vi "Parse U64 Ctl Regs.vi"(9 "NTeeths In":T5, 10 "FullyCustomTeeths In":T3, 11 "U64":T1[](array[typedef])) -> (1 "NTeeths Out":T5, 2 "FullyCustomTeeths In":T3)   [LabVIEW 2011, in "Engine Sim System Explorer.lvlib"]
uses:
  Engine Sim System Explorer.lvlib
  TypeDefs/NTeethRegs.ctl
  TypeDefs/FullyCustomRegs.ctl
  <userlib>/_FPGA Interface Advanced Tools/FPGA Bitfile Utility/TypeDefs/Scalar Register.ctl
  <userlib>/_FPGA Interface Advanced Tools/FPGA Bitfile Utility/FPGA Bitfile Utility.lvlib
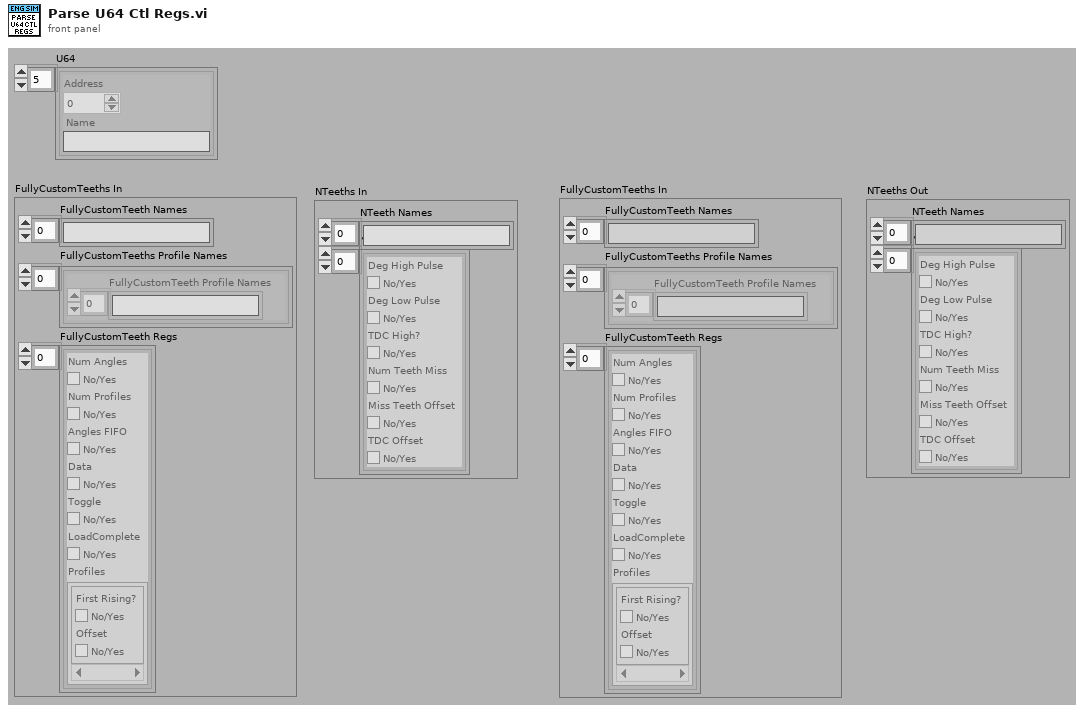
[diagram p1: front panel]
types:
  T1 = typedef "FPGA Bitfile Utility.lvlib/Scalar Register.ctl" = cluster{"Address":u32, "Name":string}
  T2 = typedef "Engine Sim System Explorer.lvlib/FullyCustomRegs.ctl" = cluster{"Num Angles":bool, "Num Profiles":bool, "Angles FIFO":bool, "Data":bool, "Toggle":bool, "LoadComplete":bool, "Profiles":cluster{"First Rising?":bool, "Offset":bool}[]}
  T3 = cluster{"FullyCustomTeeth Names":string[], "FullyCustomTeeths Profile Names":cluster{"FullyCustomTeeth Profile Names":string[]}[], "FullyCustomTeeth Regs":T2[]}
  T4 = typedef "Engine Sim System Explorer.lvlib/NTeethRegs.ctl" = cluster{"Deg High Pulse":bool, "Deg Low Pulse":bool, "TDC High?":bool, "Num Teeth Miss":bool, "Miss Teeth Offset":bool, "TDC Offset":bool}
  T5 = cluster{"NTeeth Names":string[], "NTeeth Regs":T4[]}
  T6 = cluster{"FullyCustomTeeth Profile Names":string[]}
  T7 = cluster{"FullyCustomTeeth Profile Names":string[]}[]
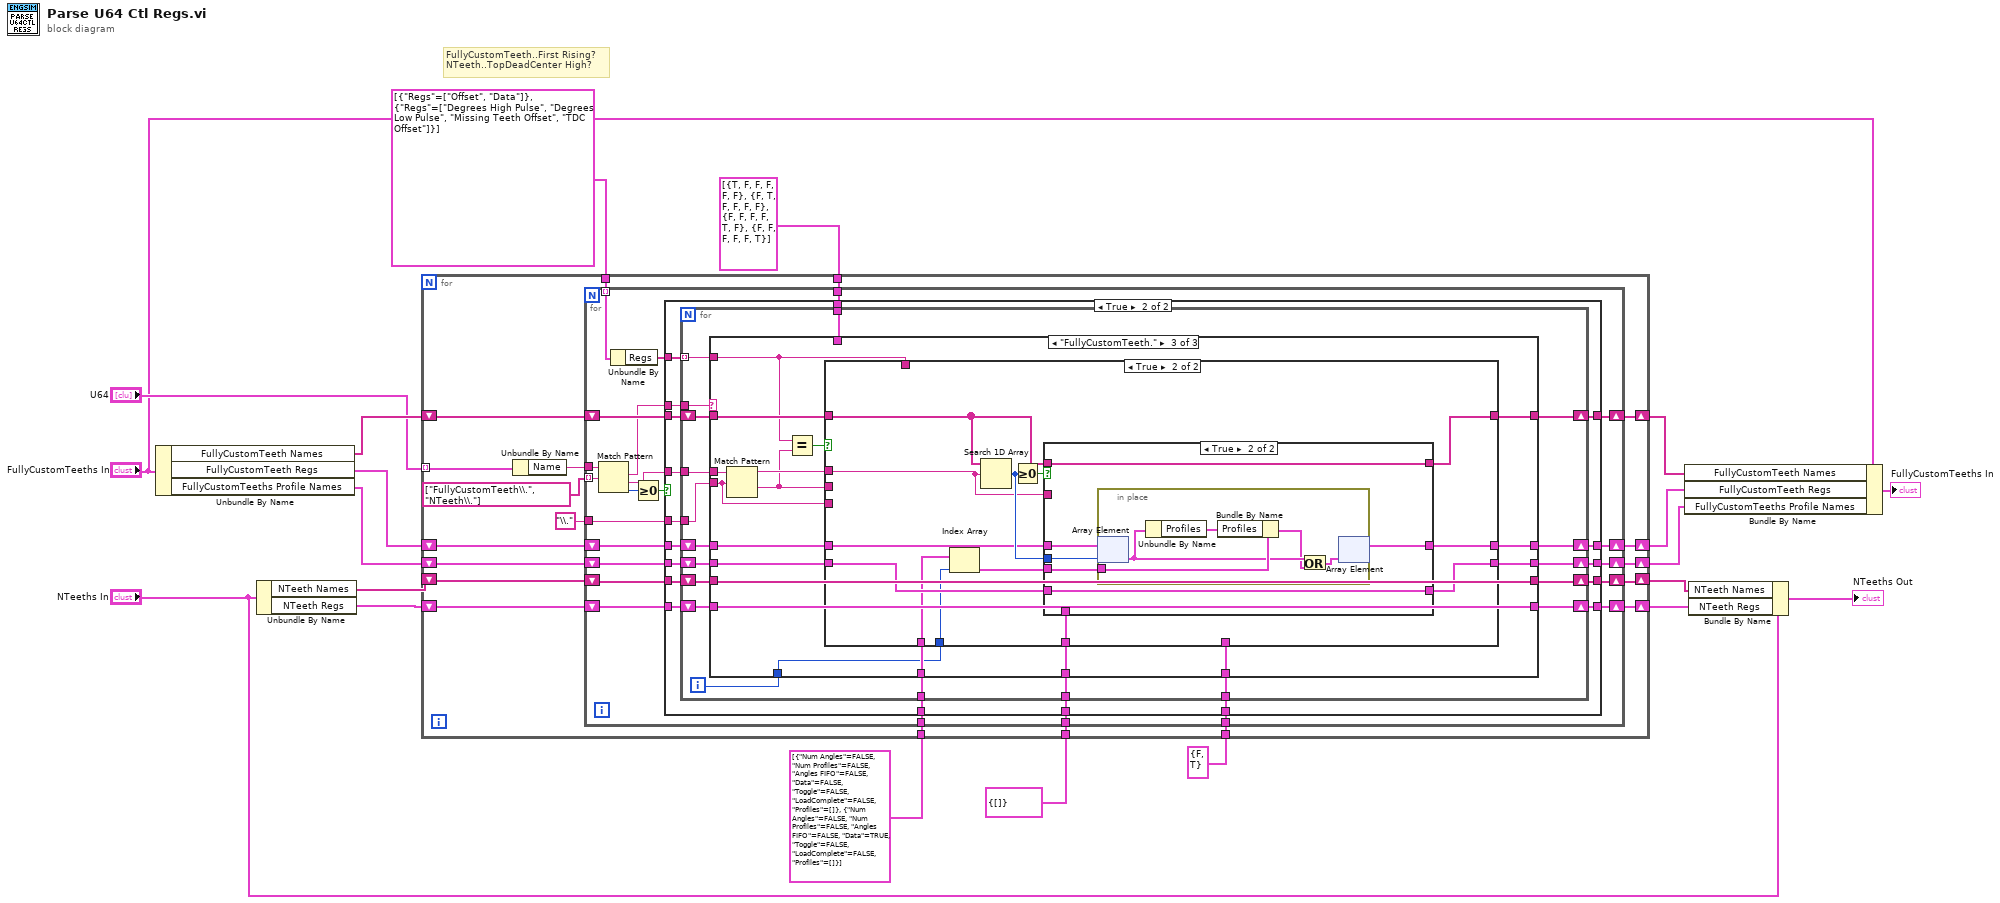
[diagram p0: block diagram]
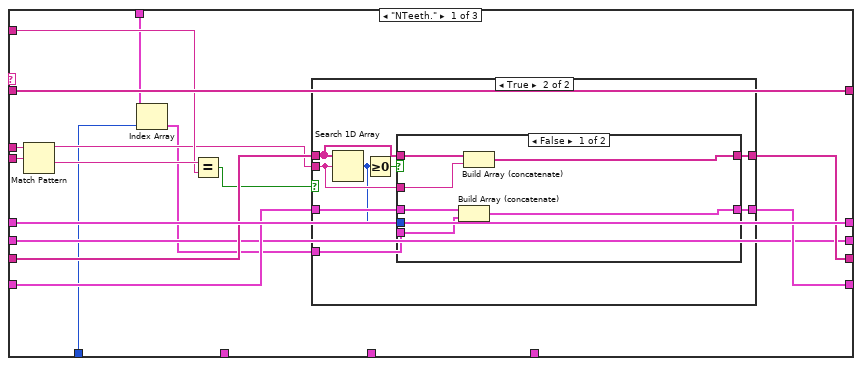
[diagram p3: hidden frame]
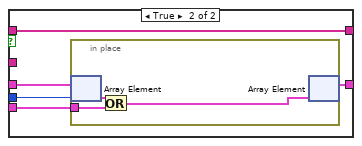
[diagram p5: hidden frame]
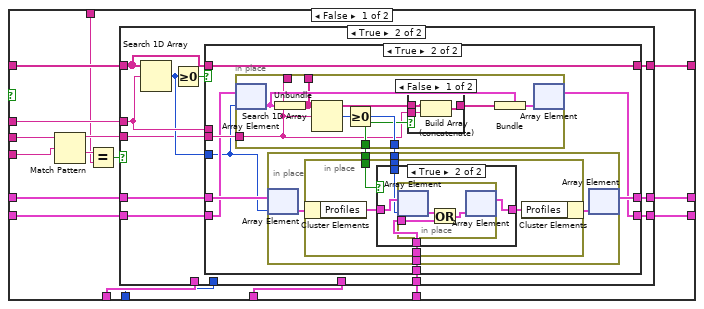
[diagram p7: hidden frame]
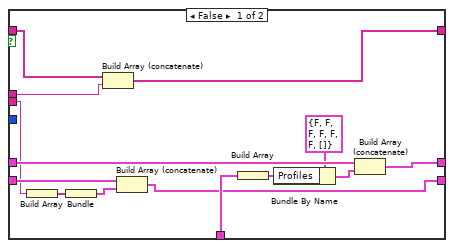
[diagram p9: hidden frame]
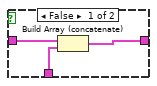
[diagram p11: hidden frame]
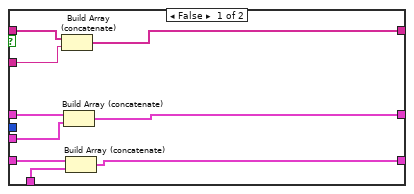
[diagram p12: hidden frame]
diagram:
  # "FullyCustomTeeth..First Rising?\nNTeeth..TopDeadCenter High?"
  n1 = Unbundle By Name("FullyCustomTeeths In") -> ("FullyCustomTeeth Names"=w12:string[], "FullyCustomTeeth Regs"=w13:T2[], "FullyCustomTeeths Profile Names"=w5:T7)
  n2 = Unbundle By Name("NTeeths In") -> ("NTeeth Names"=w14:string[], "NTeeth Regs"=w15:T4[])
  n3 = for {
    tunnel: "U64" -> [w39] mode=indexing
    tunnel: cluster{"First Rising?":bool, "Offset":bool} {"First Rising?"=FALSE, "Offset"=TRUE} ("Profile") -> [w37]
    shift-right: [w36] -> w17
    shift-left: w13 -> [w35]
    shift-right: [w34] -> w16
    shift-left: w12 -> [w33]
    tunnel: cluster{"Regs":string[]}[] [{"Regs"=["Offset", "Data"]}, {"Regs"=["Degrees High Pulse", "Degrees Low Pulse", "Missing Teeth Offset", "TDC Offset"]}] -> [w31]
    shift-right: [w30] -> w20
    shift-left: w15 -> [w29]
    tunnel: T4[] [{"Deg High Pulse"=TRUE, "Deg Low Pulse"=FALSE, "TDC High?"=FALSE, "Num Teeth Miss"=FALSE, "Miss Teeth Offset"=FALSE, "TDC Offset"=FALSE}, {"Deg High Pulse"=FALSE, "Deg Low Pulse"=TRUE, "TDC High?"=FALSE, "Num Teeth Miss"=FALSE, "Miss Teeth Offset"=FALSE, "TDC Offset"=FALSE}, {"Deg High Pulse"=FALSE, "Deg Low Pulse"=FALSE, "TDC High?"=FALSE, "Num Teeth Miss"=FALSE, "Miss Teeth Offset"=TRUE, "TDC Offset"=FALSE}, {"Deg High Pulse"=FALSE, "Deg Low Pulse"=FALSE, "TDC High?"=FALSE, "Num Teeth Miss"=FALSE, "Miss Teeth Offset"=FALSE, "TDC Offset"=TRUE}] -> [w28]
    shift-right: [w26] -> w19
    shift-left: w14 -> [w25]
    shift-right: [w23] -> w4
    shift-left: w5 -> [w24]
    tunnel: T2[] [{"Num Angles"=FALSE, "Num Profiles"=FALSE, "Angles FIFO"=FALSE, "Data"=FALSE, "Toggle"=FALSE, "LoadComplete"=FALSE, "Profiles"=[]}, {"Num Angles"=FALSE, "Num Profiles"=FALSE, "Angles FIFO"=FALSE, "Data"=TRUE, "Toggle"=FALSE, "LoadComplete"=FALSE, "Profiles"=[]}] -> [w22]
    tunnel: T6 {"FullyCustomTeeth Profile Names"=[]} ("FullyCustomTeeth") -> [w21]
    n4 = Unbundle By Name(w39) -> ("Name"=w38:string)
    n5 = for {
      tunnel: w38 -> [w62]
      tunnel: w37 -> [w58]
      tunnel: string[] ["FullyCustomTeeth\\.", "NTeeth\\."] -> [w53] mode=indexing
      shift-right: [w55] -> w34
      shift-left: w33 -> [w54]
      shift-right: [w57] -> w36
      shift-left: w35 -> [w56]
      tunnel: w31 -> [w52] mode=indexing
      shift-right: [w49] -> w30
      shift-left: w29 -> [w48]
      tunnel: w28 -> [w47]
      tunnel: "\\." ("regular expression") -> [w46]
      shift-right: [w45] -> w26
      shift-left: w25 -> [w44]
      shift-right: [w42] -> w23
      shift-left: w24 -> [w43]
      tunnel: w22 -> [w41]
      tunnel: w21 -> [w40]
      n6 = Match Pattern(string=w62, regular expression=w53) -> (match substring=w50:string, after substring=w59:string, offset past match=w61:i32)  [unwired: 1 in, 1 out]
      n7 = Unbundle By Name(w52) -> ("Regs"=w51:string[])
      n8 = Greater Or Equal To 0?(x=w61) -> (x >= 0?=w60:bool)
      n9 = case shown="True" w60 {
        tunnel: w59 -> [_ w85]
        tunnel: w58 -> [_ w84]
        tunnel: [w66 w83] -> w57
        tunnel: w56 -> [w66 w82]
        tunnel: [w67 w81] -> w55
        tunnel: w54 -> [w67 w80]
        tunnel: w51 -> [_ w79]
        tunnel: w50 -> [_ w78]
        tunnel: [w65 w77] -> w49
        tunnel: w48 -> [w65 w76]
        tunnel: w47 -> [_ w75]
        tunnel: w46 -> [_ w74]
        tunnel: [w64 w73] -> w45
        tunnel: w44 -> [w64 w72]
        tunnel: w43 -> [w63 w71]
        tunnel: [w63 w70] -> w42
        tunnel: w41 -> [_ w69]
        tunnel: w40 -> [_ w68]
        frame False {
        }
        frame True {
          n10 = for {
            tunnel: w85 -> [w93]
            tunnel: w84 -> [w104]
            shift-right: [w101] -> w81
            shift-left: w80 -> [w100]
            shift-right: [w103] -> w83
            shift-left: w82 -> [w102]
            tunnel: w79 -> [w91] mode=indexing
            tunnel: w78 -> [w99]
            shift-right: [w98] -> w77
            shift-left: w76 -> [w96]
            tunnel: w75 -> [w97]
            tunnel: w74 -> [w92]
            shift-right: [w95] -> w73
            shift-left: w72 -> [w94]
            shift-right: [w89] -> w70
            shift-left: w71 -> [w90]
            tunnel: w69 -> [w88]
            tunnel: w68 -> [w87]
            i -> [w86]
            n11 = case shown="\"FullyCustomTeeth.\"" w99 {
              tunnel: w93 -> [w113 _ w160]
              tunnel: w104 -> [_ _ w167]
              tunnel: [w119 w148 w166] -> w103
              tunnel: w102 -> [w119 w148 w165]
              tunnel: [w120 w149 w164] -> w101
              tunnel: w100 -> [w120 w149 w163]
              tunnel: [w116 w147 w162] -> w98
              tunnel: w97 -> [w107 _ _]
              tunnel: w96 -> [w115 w147 w162]
              tunnel: [w117 w146 w161] -> w95
              tunnel: w94 -> [w118 w146 w161]
              tunnel: w92 -> [w112 _ w159]
              tunnel: w91 -> [w111 _ w153]
              tunnel: w90 -> [w108 w145 w157]
              tunnel: [w108 w145 w156] -> w89
              tunnel: w88 -> [_ _ w152]
              tunnel: w87 -> [_ _ w151]
              tunnel: w86 -> [w106 _ w150]
              frame "NTeeth." {
                n12 = Match Pattern(string=w113, regular expression=w112) -> (before substring=w109:string, after substring=w114:string)  [unwired: 1 in, 2 out]
                n13 = Index Array(array=w107, index=w106) -> (element=w105:T4)
                n14 = Equal?(x=w114, y=w111) -> (x = y?=w110:bool)
                n15 = case shown="True" w110 {
                  tunnel: w109 -> [_ w126]
                  tunnel: [w121 w128] -> w116
                  tunnel: w115 -> [w121 w129]
                  tunnel: [w122 w125] -> w117
                  tunnel: w118 -> [w122 w127]
                  tunnel: w105 -> [_ w123]
                  frame False {
                  }
                  frame True {
                    n16 = Search 1D Array(1D array=w127, element=w126) -> (index of element=w124:i32)  [unwired: 1 in]
                    n17 = Greater Or Equal To 0?(x=w124) -> (x >= 0?=w130:bool)
                    n18 = case shown="False" w130 {
                      tunnel: w129 -> [w136 w140]
                      tunnel: w123 -> [w135 w138]
                      tunnel: [w134 w137] -> w128
                      tunnel: w127 -> [w133 w141]
                      tunnel: w126 -> [w132 _]
                      tunnel: [w131 w141] -> w125
                      tunnel: w124 -> [_ w139]
                      frame False {
                        n19 = Build Array (concatenate)(w136, w135) -> (w134:T4[])
                        n20 = Build Array (concatenate)(w133, w132) -> (w131:string[])
                      }
                      frame True {
                        n21 = in-place {
                          in-place-border: w138 -> [w143]
                          n22 = in-place-array #1(w140, w139) -> (w144:T4)
                          n23 = Or(x=w144, y=w143) -> (x .or. y?=w142:T4)
                          n24 = in-place-array #1(w142) -> (w137:T4[])  [unwired: 1 out]
                        }
                      }
                    }
                  }
                }
              }
              frame Default {
              }
              frame "FullyCustomTeeth." {
                n25 = Match Pattern(string=w160, regular expression=w159) -> (before substring=w158:string, after substring=w154:string)  [unwired: 1 in, 2 out]
                n26 = Equal?(x=w153, y=w154) -> (x = y?=w155:bool)
                n27 = case shown="True" w155 {
                  tunnel: w167 -> [w184 _]
                  tunnel: [w183 w258] -> w166
                  tunnel: w165 -> [w182 w261]
                  tunnel: [w181 w259] -> w164
                  tunnel: w163 -> [w180 w264]
                  tunnel: w154 -> [w179 _]
                  tunnel: w159 -> [w178 _]
                  tunnel: w158 -> [w177 w263]
                  tunnel: w153 -> [w173 _]
                  tunnel: w157 -> [w172 w262]
                  tunnel: [w171 w257] -> w156
                  tunnel: w152 -> [w170 w256]
                  tunnel: w151 -> [w168 w260]
                  tunnel: w150 -> [w169 w255]
                  frame False {
                    n28 = Match Pattern(string=w179, regular expression=w178) -> (before substring=w176:string, after substring=w174:string)  [unwired: 1 in, 2 out]
                    n29 = Equal?(x=w174, y=w173) -> (x = y?=w175:bool)
                    n30 = case shown="True" w175 {
                      tunnel: w177 -> [_ w194]
                      tunnel: w184 -> [_ w197]
                      tunnel: [w186 w196] -> w183
                      tunnel: w182 -> [w186 w198]
                      tunnel: [w187 w193] -> w181
                      tunnel: w180 -> [w187 w195]
                      tunnel: w176 -> [_ w189]
                      tunnel: w172 -> [w185 w190]
                      tunnel: [w185 w191] -> w171
                      tunnel: w170 -> [_ _]
                      tunnel: w169 -> [_ _]
                      tunnel: w168 -> [_ _]
                      frame False {
                      }
                      frame True {
                        n31 = Search 1D Array(1D array=w195, element=w194) -> (index of element=w192:i32)  [unwired: 1 in]
                        n32 = Greater Or Equal To 0?(x=w192) -> (x >= 0?=w188:bool)
                        n33 = case shown="True" w188 {
                          tunnel: w198 -> [w212 w221]
                          tunnel: w197 -> [w205 w220]
                          tunnel: [w211 w219] -> w196
                          tunnel: w195 -> [w210 w222]
                          tunnel: w194 -> [w209 _]
                          tunnel: [w208 w222] -> w193
                          tunnel: w192 -> [_ w214]
                          tunnel: [w199 w213] -> w191
                          tunnel: w190 -> [w203 w215]
                          tunnel: w189 -> [w202 w218]
                          frame False {
                            n34 = Build Array(w202) -> (w201:string[])
                            n35 = Bundle(w201) -> (w200:cluster{string[]})  [unwired: 1 in]
                            n36 = Build Array (concatenate)(w210, w209) -> (w208:string[])
                            n37 = Build Array (concatenate)(w203, w200) -> (w199:T7)
                            n38 = Build Array(w205) -> (w204:cluster{"First Rising?":bool, "Offset":bool}[])
                            n39 = Bundle By Name(cluster=T2 {"Num Angles"=FALSE, "Num Profiles"=FALSE, "Angles FIFO"=FALSE, "Data"=FALSE, "Toggle"=FALSE, "LoadComplete"=FALSE, "Profiles"=[]} ("element"), "Profiles"=w204) -> (w207:T2)
                            n40 = Build Array (concatenate)(w212, w207) -> (w211:T2[])
                          }
                          frame True {
                            n41 = in-place {
                              in-place-border: w218 -> [w223]
                              in-place-border: [w225] -> w217
                              in-place-border: [w229] -> w216
                              in-place-border: [w224] -> _
                              in-place-border: [w223] -> _
                              n42 = in-place-array #2(w215, w214) -> (w228:T6)
                              n43 = Unbundle(w228) -> ("FullyCustomTeeth Profile Names"=w224:string[])
                              n44 = Search 1D Array(1D array=w224, element=w223) -> (index of element=w229:i32)  [unwired: 1 in]
                              n45 = Greater Or Equal To 0?(x=w229) -> (x >= 0?=w225:bool)
                              n46 = case shown="False" w225 {
                                tunnel: w224 -> [w232 w233]
                                tunnel: [w231 w233] -> w226
                                tunnel: w223 -> [w230 _]
                                frame False {
                                n47 = Build Array (concatenate)(w232, w230) -> (w231:string[])
                                }
                                frame True {
                                }
                              }
                              n48 = Bundle(cluster=w228, "FullyCustomTeeth Profile Names"=w226) -> (w227:T6)
                              n49 = in-place-array #2(w227) -> (w213:T7)  [unwired: 1 out]
                            }
                            n50 = in-place {
                              in-place-border: w220 -> [w238]
                              in-place-border: w217 -> [w235]
                              in-place-border: w216 -> [w234]
                              n51 = in-place-array #3(w221, w214) -> (w237:T2)
                              n52 = in-place {
                                in-place-border: w238 -> [w243]
                                in-place-border: w235 -> [w240]
                                in-place-border: w234 -> [w239]
                                n53 = in-place-cluster #4(w237) -> ("Profiles"=w242:cluster{"First Rising?":bool, "Offset":bool}[])
                                n54 = case shown="True" w240 {
                                tunnel: w243 -> [w245 w250]
                                tunnel: w242 -> [w246 w249]
                                tunnel: [w244 w248] -> w241
                                tunnel: w239 -> [_ w247]
                                frame False {
                                n55 = Build Array (concatenate)(w246, w245) -> (w244:cluster{"First Rising?":bool, "Offset":bool}[])
                                }
                                frame True {
                                n56 = in-place {
                                in-place-border: w250 -> [w253]
                                n57 = in-place-array #5(w249, w247) -> (w251:cluster{"First Rising?":bool, "Offset":bool})
                                n58 = Or(x=w251, y=w253) -> (x .or. y?=w252:cluster{"First Rising?":bool, "Offset":bool})
                                n59 = in-place-array #5(w252) -> (w248:cluster{"First Rising?":bool, "Offset":bool}[])  [unwired: 1 out]
                                }
                                }
                                }
                                n60 = in-place-cluster #4("Profiles"=w241) -> (w236:T2)
                              }
                              n61 = in-place-array #3(w236) -> (w219:T2[])  [unwired: 1 out]
                            }
                          }
                        }
                      }
                    }
                  }
                  frame True {
                    n62 = Index Array(array=w256, index=w255) -> (element=w254:T2)
                    n63 = Search 1D Array(1D array=w264, element=w263) -> (index of element=w265:i32)  [unwired: 1 in]
                    n64 = Greater Or Equal To 0?(x=w265) -> (x >= 0?=w266:bool)
                    n65 = case shown="True" w266 {
                      tunnel: w261 -> [w275 w280]
                      tunnel: w254 -> [w274 w278]
                      tunnel: [w273 w277] -> w258
                      tunnel: w264 -> [w272 w281]
                      tunnel: w263 -> [w271 _]
                      tunnel: [w270 w281] -> w259
                      tunnel: w265 -> [_ w279]
                      tunnel: w262 -> [w269 w276]
                      tunnel: [w268 w276] -> w257
                      tunnel: w260 -> [w267 _]
                      frame False {
                        n66 = Build Array (concatenate)(w272, w271) -> (w270:string[])
                        n67 = Build Array (concatenate)(w275, w274) -> (w273:T2[])
                        n68 = Build Array (concatenate)(w269, w267) -> (w268:T7)
                      }
                      frame True {
                        n69 = in-place {
                          in-place-border: w278 -> [w285]
                          n70 = in-place-array #6(w280, w279) -> (w284:T2)
                          n71 = Unbundle By Name(w284) -> ("Profiles"=w283:cluster{"First Rising?":bool, "Offset":bool}[])
                          n72 = Bundle By Name(cluster=w285, "Profiles"=w283) -> (w282:T2)
                          n73 = Or(x=w284, y=w282) -> (x .or. y?=w286:T2)
                          n74 = in-place-array #6(w286) -> (w277:T2[])  [unwired: 1 out]
                        }
                      }
                    }
                  }
                }
              }
            }
          }
        }
      }
    }
  }
  n75 = Bundle By Name(cluster="FullyCustomTeeths In", "FullyCustomTeeth Names"=w16, "FullyCustomTeeth Regs"=w17, "FullyCustomTeeths Profile Names"=w4) -> (→"FullyCustomTeeths In":T3)
  n76 = Bundle By Name(cluster="NTeeths In", "NTeeth Names"=w19, "NTeeth Regs"=w20) -> (→"NTeeths Out":T5)
